vi "CS-4 Config.vi"(5 "limits":T1={"Lower Current Limit"=-10.0, "Upper Current Limit"=10.0, "Voltage Limit"=5.0} {"Voltage Limit" min=0.0 max=5.0 format="%.2f"; "Upper Current Limit" min=-100.0 max=100.0 format="%.2f"; "Lower Current Limit" min=-100.0 max=100.0 format="%.1f"}, 7 "Units":enum16{"Amps", "Kilogauss", "Tesla"}(ring), 8 "error in (no error)":errorcluster, 9 "sweep rates":T2={"rate 0"=0.5, "rate 1"=0.25, "rate 2"=0.125, "rate 3"=10.0} {"rate 3" min=0.0001 max=99.8 format="%.4f"; "rate 2" min=0.0001 max=99.8 format="%.4f"; "rate 1" min=0.0001 max=99.8 format="%.4f"; "rate 0" min=0.0001 max=99.8 format="%.4f"}, 10 "sweep range":cluster{"range 0":dbl, "range 1":dbl}={"range 0"=60.0, "range 1"=85.0} {"range 1" format="%.3f"; "range 0" format="%.3f"}, 11 "VISA session":refnum<visa-resource-name>) -> (0 "error out":errorcluster={"status"=TRUE, "code"=0, "source"=""}, 3 "dup VISA session":refnum<visa-resource-name>)   [LabVIEW 2016]
doc: "CS-4 Config.vi uses the CS-4 driver VI's to configure a CS-4 Magnet Power Supply with remotely selectable parameters. This information includes display units, sweep limits, and voltage limits.\n\nA VISA channel must be opened using CS-4 Initialize.vi before this VI is invoked."
panel:
  in  "Cancel":bool
  in  "Send":bool
  out "max supply current":dbl=100.0 format="%.3f"
  out "range 2 start":dbl format="%.3f"
  out "range 1 start":dbl format="%.3f"
  out "Cryo Logo":bool
  # "CRYOMAGNETICS, INC."
  # "Model CS-4"
  # "Magnet Power Supply Configure"
  # "Sweep Rates"
  # "Range 1"
  # "0.000"
  # "TO"
  # "Range 2"
  # "TO"
  # "Range 3"
  # "TO"
  # "Fast Mode"
  # "Limits"
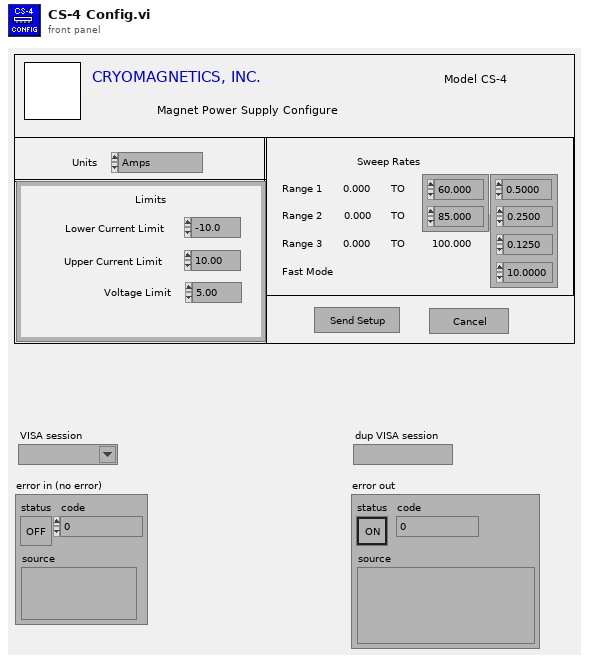
[diagram p1: front panel]
types:
  T1 = cluster{"Lower Current Limit":dbl, "Upper Current Limit":dbl, "Voltage Limit":dbl}
  T2 = cluster{"rate 0":dbl, "rate 1":dbl, "rate 2":dbl, "rate 3":dbl}
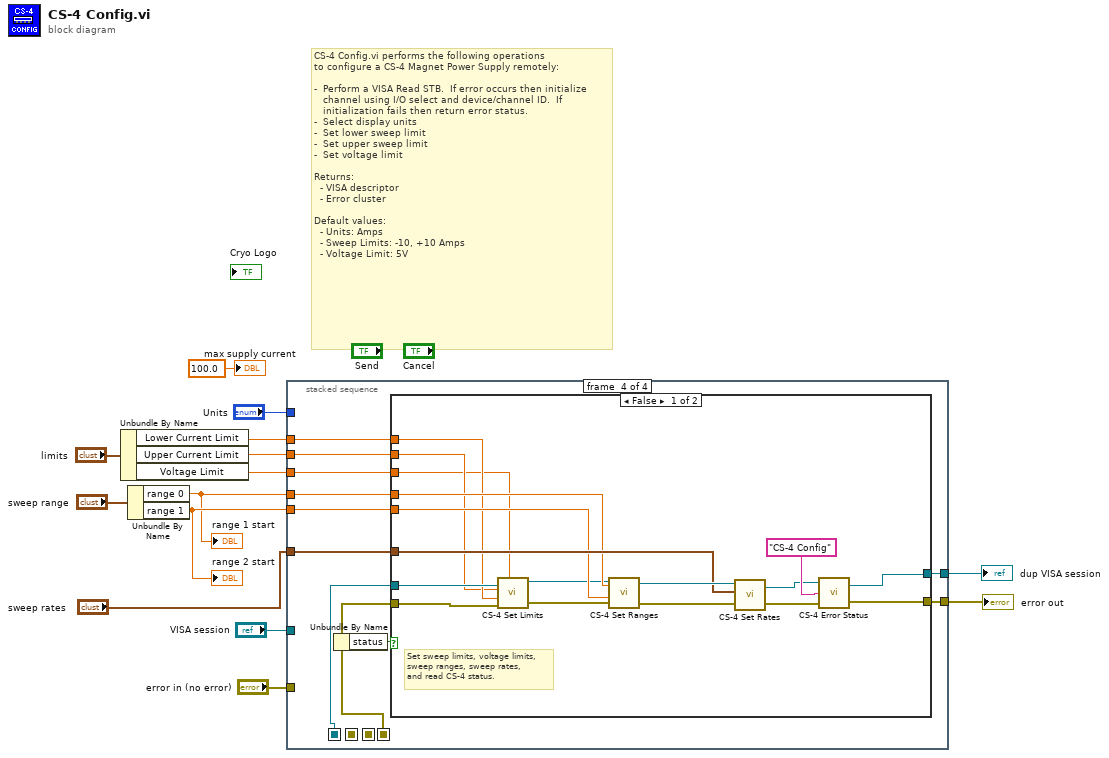
[diagram p0: block diagram]
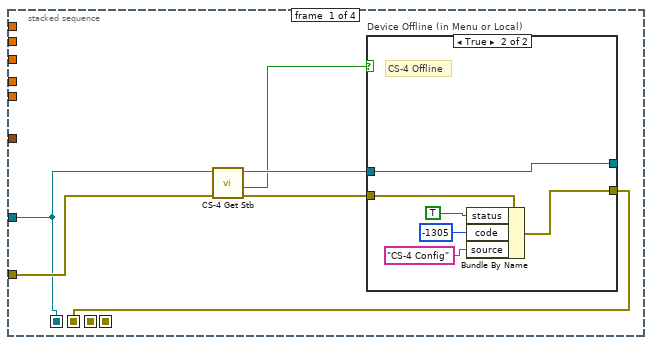
[diagram p2: hidden frame]
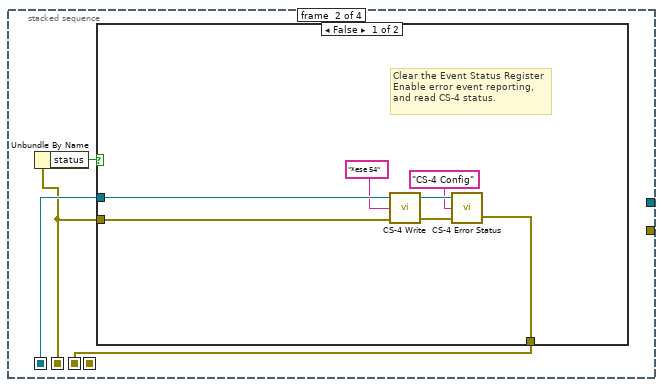
[diagram p4: hidden frame]
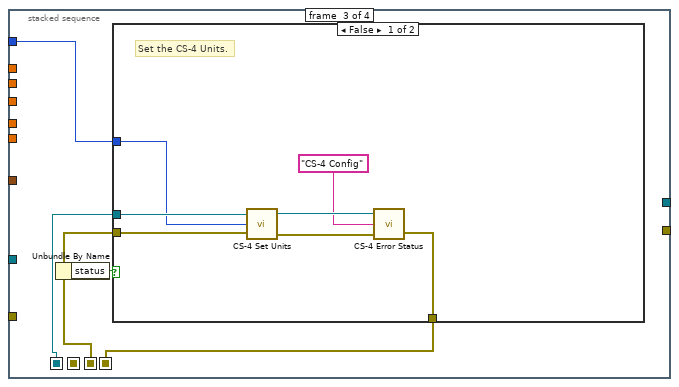
[diagram p6: hidden frame]
diagram:
  # "CS-4 Config.vi performs the following operations\nto configure a CS-4 Magnet Power Supply remotely:\n\n-  Perform a VISA Read STB.  If error occurs then initialize \n   channel using I/O select and device/channel ID.  If \n   initialization fails then return error status.\n-  Select display units\n-  Set lower sweep limit\n-  Set upper sweep limit\n-  Set voltage limit\n\nReturns:\n  - VISA descriptor\n  - Error cluster\n\nDefault values:\n  - Units: Amps\n  - Sweep Limits: -10, +10 Amps\n  - Voltage Limit: 5V"
  n1 = Unbundle By Name("limits") -> ("Lower Current Limit"=w8:dbl, "Upper Current Limit"=w7:dbl, "Voltage Limit"=w6:dbl)
  n2 = Unbundle By Name("sweep range") -> ("range 0"=w2:dbl, "range 1"=w3:dbl)
  "range 1 start" <- w2
  "range 2 start" <- w3
  n3 = stacked-sequence {
    seq-local: [_ w29 _ _] -> [_ _ w42 _]
    seq-local: [w18 _ _ _] -> [_ w31 w44 w62]
    seq-local: [_ _ w41 _] -> [_ _ _ w61]
    seq-local: [w20 _ _ _] -> [_ w30 _ _]
    tunnel: "error in (no error)" -> [w19 _ _ _]
    tunnel: "Units" -> [_ _ w43 _]
    tunnel: w8 -> [_ _ _ w63]
    tunnel: [_ _ _ w58] -> w12
    tunnel: [_ _ _ w57] -> w11
    tunnel: "VISA session" -> [w18 _ _ _]
    tunnel: w7 -> [_ _ _ w60]
    tunnel: w6 -> [_ _ _ w59]
    tunnel: w2 -> [_ _ _ w56]
    tunnel: w3 -> [_ _ _ w55]
    tunnel: "sweep rates" -> [_ _ _ w54]
    frame #0 {
      n4 = call "CS-4 Get Stb.vi"("error in (no error)"=w19, "VISA session"=w18) -> ("error out"=w17:errorcluster, "Off Line"=w15:bool, "dup VISA session"=w16:refnum<visa-resource-name>)  [unwired: 2 in, 1 out]
      n5 = case "Device Offline (in Menu or Local)" shown="True" w15 {
        tunnel: [w22 w26] -> _
        tunnel: w16 -> [w22 w26]
        tunnel: [w21 w27] -> w20
        tunnel: w17 -> [w21 w28]
        frame False {
          # "CS-4 not offline"
        }
        frame True {
          # "CS-4 Offline"
          n6 = Bundle By Name(cluster=w28, "status"=TRUE, "code"=-1305, "source"="CS-4 Config") -> (w27:errorcluster)
        }
      }
    }
    frame #1 {
      n7 = Unbundle By Name(w30) -> ("status"=w32:bool)
      n8 = case shown="False" w32 {
        tunnel: w30 -> [w34 w40]
        tunnel: w31 -> [w35 _]
        tunnel: [w37 w40] -> w29
        frame False {
          # "Clear the Event Status Register\nEnable error event reporting,\nand read CS-4 status."
          n9 = call "CS-4 Write.vi"("error in (no error)"=w34, "write buffer (\"\")"="*ese 54", "VISA session"=w35) -> ("error out"=w38:errorcluster, "dup VISA session"=w39:refnum<visa-resource-name>)  [unwired: 1 out]
          n10 = call "CS-4 Error Status.vi"("error in (no error)"=w38, "VI name"="CS-4 Config", "VISA session"=w39) -> ("error out"=w37:errorcluster)  [unwired: 1 out]
        }
        frame True {
        }
      }
    }
    frame #2 {
      n11 = Unbundle By Name(w42) -> ("status"=w45:bool)
      n12 = case shown="False" w45 {
        tunnel: w42 -> [w52 w53]
        tunnel: w44 -> [w51 _]
        tunnel: w43 -> [w46 _]
        tunnel: [w48 w53] -> w41
        frame False {
          # "Set the CS-4 Units."
          n13 = call "CS-4 Set Units.vi"("error in (no error)"=w52, "units"=w46, "VISA session"=w51) -> ("error out"=w49:errorcluster, "dup VISA session"=w50:refnum<visa-resource-name>)  [unwired: 1 in]
          n14 = call "CS-4 Error Status.vi"("error in (no error)"=w49, "VI name"="CS-4 Config", "VISA session"=w50) -> ("error out"=w48:errorcluster)  [unwired: 1 out]
        }
        frame True {
        }
      }
    }
    frame #3 {
      n15 = Unbundle By Name(w61) -> ("status"=w64:bool)
      n16 = case shown="False" w64 {
        tunnel: w61 -> [w81 w83]
        tunnel: w62 -> [w80 w82]
        tunnel: w63 -> [w67 _]
        tunnel: [w73 w83] -> w58
        tunnel: w60 -> [w66 _]
        tunnel: w59 -> [w65 _]
        tunnel: [w71 w82] -> w57
        tunnel: w56 -> [w70 _]
        tunnel: w55 -> [w69 _]
        tunnel: w54 -> [w72 _]
        frame False {
          # "Set sweep limits, voltage limits,\nsweep ranges, sweep rates, \nand read CS-4 status."
          n17 = call "CS-4 Set Limits.vi"("voltage limit"=w65, "error in (no error)"=w81, "lower limit"=w67, "upper limit"=w66, "VISA session"=w80) -> ("error out"=w79:errorcluster, "dup VISA session"=w68:refnum<visa-resource-name>)  [unwired: 2 in]
          n18 = call "CS-4 Set Ranges.vi"("error in (no error)"=w79, "range 1"=w69, "range 0"=w70, "VISA session"=w68) -> ("error out"=w77:errorcluster, "dup VISA session"=w78:refnum<visa-resource-name>)
          n19 = call "CS-4 Set Rates.vi"("error in (no error)"=w77, "sweep rates"=w72, "VISA session"=w78) -> ("error out"=w75:errorcluster, "dup VISA session"=w74:refnum<visa-resource-name>)  [unwired: 1 in]
          n20 = call "CS-4 Error Status.vi"("error in (no error)"=w75, "VI name"="CS-4 Config", "VISA session"=w74) -> ("error out"=w73:errorcluster, "dup VISA session"=w71:refnum<visa-resource-name>)
        }
        frame True {
        }
      }
    }
  }
  "error out" <- w12
  "dup VISA session" <- w11
  "max supply current" <- 100.0 ("max supply current")
